vi "runtime io test.vi"() -> ()   [LabVIEW 2013, in "scan engine tests.lvlib"]
uses:
  scan engine tests.lvlib
  execution/Scan Engine runtime.lvclass
  <vilib>/NI/Tag Bus/tag/tag descriptor.lvclass/tag descriptor.ctl
  <vilib>/NI/Tag Bus/table/data polymorphs/write one/write Double.vi
  <vilib>/NI/Tag Bus/table/data polymorphs/read one/read Double.vi
  <vilib>/NI/Tag Bus/tag/read tag name.vi
  <vilib>/NI/Tag Bus/tag/read data type.vi
  <vilib>/NI/Tag Bus/dictionary/data dictionary.lvclass
  <vilib>/NI/Tag Bus/table/data table.lvlib
  <vilib>/NI/Tag Bus Module Framework/channel/TBM channel.lvclass
panel:
  out "inputs changed?":bool
  out "no error":errorcluster
  # "This is expected to remain false until you write code for input"
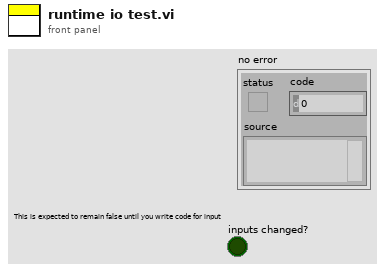
[diagram p1: front panel]
types:
  T1 = typedef "tag bus.lvlib/tag descriptor.lvclass/Data Type.ctl" = enum16{"Double", "Single", "I64", "I32", "I16", "I8", "U64", "U32", "U16", "U8", "Boolean", "String", "Array of Double", "Array of Single", "Array of I64", "Array of I32", "Array of I16", "Array of I8", "Array of U64", "Array of U32", "Array of U16", "Array of U8", "Array of Boolean", "Array of String"}
  T2 = typedef "TBM channel.lvclass/data tables.ctl" = cluster{"input data":T3, "processing parameter":T3, "processing result":T3, "output data":T3}
  T3 = typedef "tag bus.lvlib/dictionary table pair.ctl" = cluster{"data dictionary":refnum<class "data dictionary.lvclass">, "data table":T4}
  T4 = typedef "tag bus.lvlib/data table.lvlib/data table.ctl" = cluster{"Double":dbl[], "Single":sgl[], "I64":i64[], "I32":i32[], "I16":i16[], "I8":i8[], "U64":u64[], "U32":u32[], "U16":u16[], "U8":u8[], "Boolean":bool[], "String":string[], "Array of Double":cluster{"DBL Array":dbl[]}[], "Array of Single":cluster{"SGL Array":sgl[]}[], "Array of I64":cluster{"I64 Array":i64[]}[], "Array of I32":cluster{"I32 Array":i32[]}[], "Array of I16":cluster{"I16 Array":i16[]}[], "Array of I8":cluster{"I8 Array":i8[]}[], "Array of U64":cluster{"U64 Array":u64[]}[], "Array of U32":cluster{"U32 Array":u32[]}[], "Array of U16":cluster{"U16 Array":u16[]}[], "Array of U8":cluster{"U8 Array":u8[]}[], "Array of Boolean":cluster{"Boolean Array":bool[]}[], "Array of String":cluster{"String Array":string[]}[]}
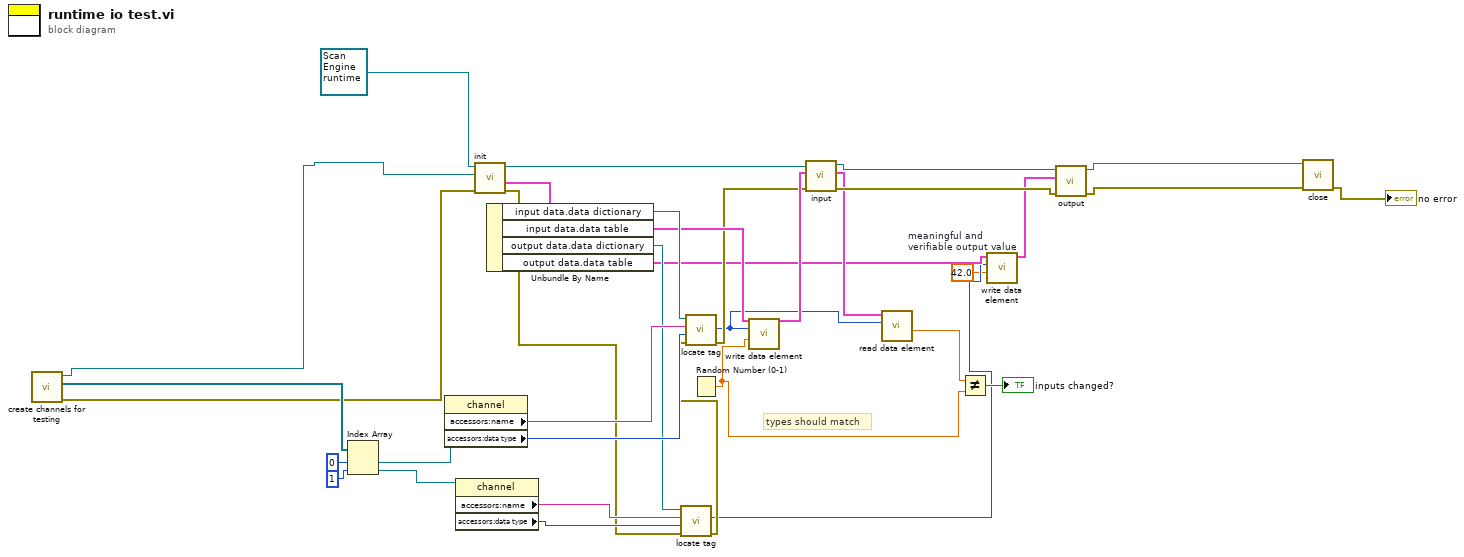
[diagram p0: block diagram]
diagram:
  w5 = 42.0  # meaningful and verifiable output value
  # "types should match"
  n1 = call "create channels for testing.vi"() -> ("error out"=w1:errorcluster, "chans"=w3:refnum<class "TBM channel.lvclass">[], "Scan Engine configuration out"=w2:refnum<class "Scan Engine configuration.lvclass">)  [unwired: 7 in, 2 out]
  n2 = Index Array(array=w3, index #1=0 ("index (row)"), index #2=1 ("index (row)")) -> (element #1=w25:refnum<class "TBM channel.lvclass">, element #2=w14:refnum<class "TBM channel.lvclass">)
  n3 = property class="channel"(reference=w25) -> ("accessors:name"=w23:string, "accessors:data type"=w24:T1)  [unwired: 1 in, 2 out]
  n4 = property class="channel"(reference=w14) -> ("accessors:name"=w12:string, "accessors:data type"=w11:T1)  [unwired: 1 in, 2 out]
  n5 = call-dynamic "init.vi"("error in"=w1, "TBM module configuration in"=w2, "Scan Engine runtime in"=refnum<class "Scan Engine runtime.lvclass"> refnum ("Scan Engine runtime")) -> ("error out"=w10:errorcluster, "data allocations"=w27:T2, "Scan Engine runtime out"=w28:refnum<class "Scan Engine runtime.lvclass">)  [unwired: 5 in, 1 out]
  n6 = Unbundle By Name(w27) -> ("input data.data dictionary"=w26:refnum<class "data dictionary.lvclass">, "input data.data table"=w22:T4, "output data.data dictionary"=w13:refnum<class "data dictionary.lvclass">, "output data.data table"=w8:T4)
  n7 = call <vilib>:"locate tag.vi"("error in"=w10, "data type"=w11, "name"=w12, "data dictionary in"=w13) -> ("error out"=w9:errorcluster, "index"=w6:i32)  [unwired: 5 in, 1 out]
  n8 = call <vilib>:"locate tag.vi"("error in"=w9, "data type"=w24, "name"=w23, "data dictionary in"=w26) -> ("error out"=w20:errorcluster, "index"=w18:i32)  [unwired: 5 in, 1 out]
  n9 = Random Number (0-1)() -> (number: 0 to 1=w17:dbl)
  n10 = call-poly <vilib>:"write data element.vi"("value"=w17, "index"=w18, "data table in"=w22) -> ("data table out"=w21:T4)  [unwired: 8 in]
  n11 = call-dynamic "input.vi"("error in"=w20, "data table in"=w21, "Scan Engine runtime in"=w28) -> ("error out"=w29:errorcluster, "data table out"=w19:T4, "Scan Engine runtime out"=w30:refnum<class "Scan Engine runtime.lvclass">)  [unwired: 6 in]
  n12 = call-poly <vilib>:"read data element.vi"("index"=w18, "data table in"=w19) -> ("value"=w16:dbl)  [unwired: 8 in, 1 out]
  n13 = Not Equal?(x=w16, y=w17) -> (x != y?=→"inputs changed?":bool)
  n14 = call-poly <vilib>:"write data element.vi"("value"=w5, "index"=w6, "data table in"=w8) -> ("data table out"=w7:T4)  [unwired: 8 in]
  n15 = call-dynamic "output.vi"("error in"=w29, "data table in"=w7, "Scan Engine runtime in"=w30) -> ("error out"=w31:errorcluster, "Scan Engine runtime out"=w32:refnum<class "Scan Engine runtime.lvclass">)  [unwired: 6 in, 1 out]
  n16 = call-dynamic "close.vi"("error in"=w31, "Scan Engine runtime in"=w32) -> ("error out"=→"no error":errorcluster)  [unwired: 9 in]
